vi "FT10_Fornax Send MonopolarCommand.vi"(8 "error in":errorcluster, 10 "Set Monopolar Command Cluster in":T4={"Serial Number"="CAMM_INTERNAL_GENERIC", "EnergyChannelID"=enum."EC_MONO_1", "CutMode"=enum."SPRAY_MODE", "CoagMode"=enum."SPRAY_MODE", "CutPowerCommand"=enum."POWER_NO_CHANGE", "CoagPowerCommand"=enum."POWER_NO_CHANGE", "Fornax Set Monopolar Command"=FALSE}, 11 "Message Handling Cluster in":T1) -> (0 "error out":errorcluster, 2 "Set Monopolar Command Cluster out":T4={"Serial Number"="CAMM_INTERNAL_GENERIC", "EnergyChannelID"=enum."EC_MONO_1", "CutMode"=enum."SPRAY_MODE", "CoagMode"=enum."SPRAY_MODE", "CutPowerCommand"=enum."POWER_NO_CHANGE", "CoagPowerCommand"=enum."POWER_NO_CHANGE", "Fornax Set Monopolar Command"=FALSE}, 3 "Message Handling Cluster out":T1)   [LabVIEW 2024]
uses:
  Controls/Control_Fornax Set Monopolar Command - Coag Power Command Enum.ctl
  Controls/Control_Fornax Set Monopolar Command - Cut Power Command Enum.ctl
  Controls/Control_Fornax Set Monopolar Command - Coag Mode Enum.ctl
  Controls/Control_Fornax Set Monopolar Command - Cut Mode Enum.ctl
  Controls/Control_Fornax Set Monopolar Command - Energy Channel ID Enum.ctl
  Controls/Control_Fornax Set Monopolar Command - Serial Number String.ctl
  Controls/Control_Fornax Set Monopolar Command Bool.ctl
  Controls/Control_Fornax Set Monopolar Command Cluster.ctl
  Controls/Control_M4X Connection.ctl
  Controls/Control_PXI-7854R FPGA Reference.ctl
  Controls/Control_Message Handling Cluster.ctl
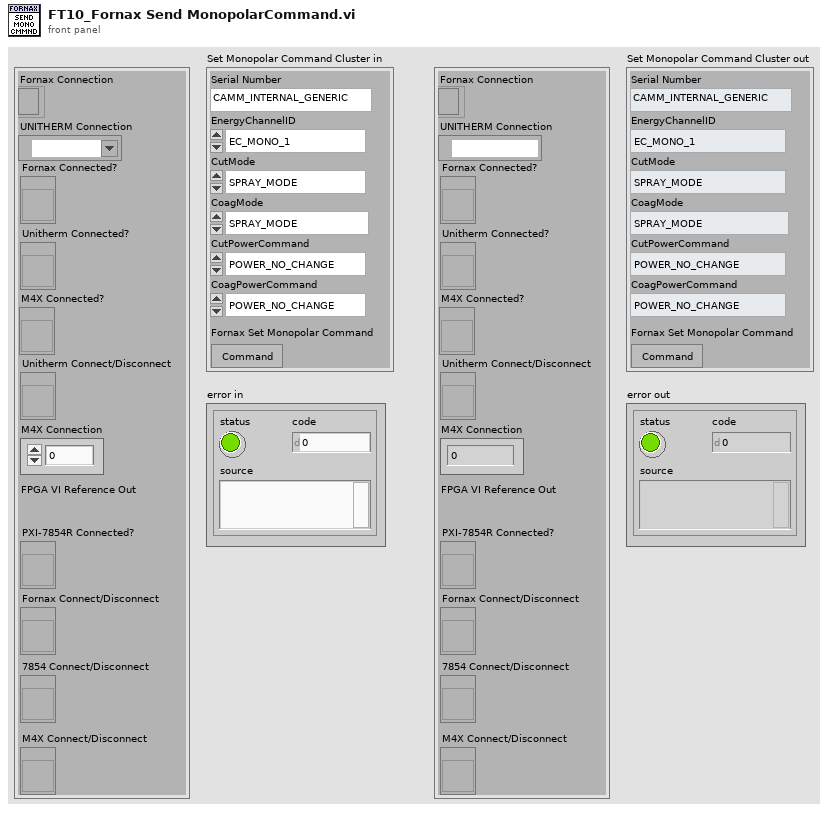
[diagram p1: front panel]
types:
  T1 = typedef "Control_Message Handling Cluster.ctl" = cluster{"Fornax Connected?":refnum<vi>, "Unitherm Connected?":refnum<vi>, "M4X Connected?":refnum<vi>, "Unitherm Connect/Disconnect":refnum<vi>, "Fornax Connection":refnum<k5>, "UNITHERM Connection":refnum<visa-resource-name>, "M4X Connection":T2, "PXI-7854R FPGA Reference":T3, "PXI-7854R Connected?":refnum<vi>, "Fornax Connect/Disconnect":refnum<vi>, "7854 Connect/Disconnect":refnum<vi>, "M4X Connect/Disconnect":refnum<vi>}
  T2 = typedef "Control_M4X Connection.ctl" = u32
  T3 = typedef "Control_PXI-7854R FPGA Reference.ctl" = refnum<k20>
  T4 = typedef "Control_Fornax Set Monopolar Command Cluster.ctl" = cluster{"Serial Number":T5, "EnergyChannelID":T6, "CutMode":T7, "CoagMode":T8, "CutPowerCommand":T9, "CoagPowerCommand":T10, "Fornax Set Monopolar Command":T11}
  T5 = typedef "Control_Fornax Set Monopolar Command - Serial Number String.ctl" = string
  T6 = typedef "Control_Fornax Set Monopolar Command - Energy Channel ID Enum.ctl" = enum16{"EC_MONO_1", "EC_BIPOLAR", "EC_MONO_2", "EC_ADVANCED", "NUM_ENERGY_CHANNELS", "EC_NOT_USED"}
  T7 = typedef "Control_Fornax Set Monopolar Command - Cut Mode Enum.ctl" = enum16{"SPRAY_MODE", "CUT_MODE", "BLEND_MODE", "FULGERATE_MODE", "BIPOLAR_MODE", "VESSEL_SEALING_MODE", "VALLEYLAB_MODE", "BIPOLAR_RESECTION_CUT_MODE", "BIPOLAR_RESECTION_COAG_MODE", "AUTOBIPOLAR_MODE", "VIPER_HLA", "SOFT_COAG_MODE", "NUM_ENERGY_MODES"}
  T8 = typedef "Control_Fornax Set Monopolar Command - Coag Mode Enum.ctl" = enum16{"SPRAY_MODE", "CUT_MODE", "BLEND_MODE", "FULGERATE_MODE", "BEPOLAR_MODE", "VESSEL_SEALING_MODE", "VALLEYLAB_MODE", "BIPOLAR_RESECTION_CUT_MODE", "BIPOLAR_RESECTION_COAG_MODE", "AUTOBIPOLAR_MODE", "VIPER_HLA", "SOFT_COAG_MODE", "NUM_ENERGY_MODES"}
  T9 = typedef "Control_Fornax Set Monopolar Command - Cut Power Command Enum.ctl" = enum16{"POWER_NO_CHANGE", "POWER_INCREASE", "POWER_DECREASE", "POWER_INCREASE_REPEAT", "POWER_DECREASE_REPEAT"}
  T10 = typedef "Control_Fornax Set Monopolar Command - Coag Power Command Enum.ctl" = enum16{"POWER_NO_CHANGE", "POWER_INCREASE", "POWER_DECREASE", "POWER_INCREASE_REPEAT", "POWER_DECREASE_REPEAT"}
  T11 = typedef "Control_Fornax Set Monopolar Command Bool.ctl" = bool
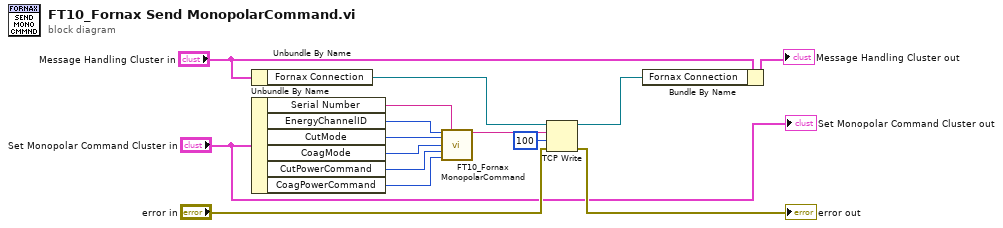
[diagram p0: block diagram]
diagram:
  n1 = Unbundle By Name("Message Handling Cluster in") -> ("Fornax Connection"=w3:refnum<k5>)
  n2 = Unbundle By Name("Set Monopolar Command Cluster in") -> ("Serial Number"=w14:T5, "EnergyChannelID"=w13:T6, "CutMode"=w12:T7, "CoagMode"=w9:T8, "CutPowerCommand"=w10:T9, "CoagPowerCommand"=w11:T10)
  n3 = call "FT10_Fornax MonopolarCommand.vi"("EnergyChannelID"=w13, "Serial Number"=w14, "CutMode"=w12, "CoagMode"=w9, "CutPowerCommand"=w10, "CoagPowerCommand"=w11) -> ("JSON Command"=w8:string)  [unwired: 9 in]
  n4 = TCP Write(connection ID=w3, data in=w8, error in (no error)="error in", 9:100 ("timeout ms (25000)")) -> (connection ID out=w1:refnum<k5>, error out=→"error out":errorcluster)  [unwired: 1 out]
  n5 = Bundle By Name(cluster="Message Handling Cluster in", "Fornax Connection"=w1) -> (→"Message Handling Cluster out":T1)
  "Set Monopolar Command Cluster out" <- "Set Monopolar Command Cluster in"
